vi "DQtoABC_noSine_src.vi"(5 "sinx":sgl, 7 "cosx":sgl, 10 "quadrature":sgl format="%#_30g", 11 "direct":sgl format="%#_30g") -> (1 "C":sgl, 2 "B":sgl, 3 "A":sgl format="%#_32g", 4 "beta":sgl format="%#_30g", 6 "alpha":sgl format="%#_30g")   [LabVIEW 2015]
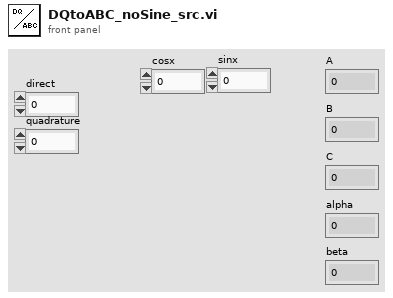
[diagram p1: front panel]
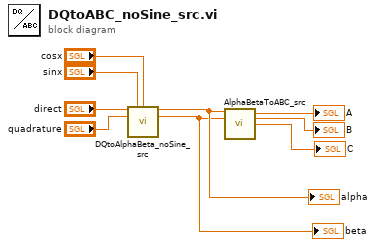
[diagram p0: block diagram]
diagram:
  n1 = call "DQtoAlphaBeta_noSine_src.vi"("direct"="direct", "sinx"="sinx", "cosx"="cosx", "quadrature"="quadrature") -> ("alpha"=w6:sgl, "beta"=w5:sgl)  [unwired: 10 in]
  "alpha" <- w6
  "beta" <- w5
  n2 = call "AlphaBetaToABC_src.vi"("alpha"=w6, "beta"=w5) -> ("A"=→"A":sgl, "B"=→"B":sgl, "C"=→"C":sgl)  [unwired: 11 in]
